vi "length_add_one.vi"(8 "error in (no error)":errorcluster, 11 "DoublyLinkedList in":refnum<class "DoublyLinkedList.lvclass">) -> (0 "error out":errorcluster, 3 "DoublyLinkedList out":refnum<class "DoublyLinkedList.lvclass">)   [LabVIEW 2021, in "DoublyLinkedList.lvclass"]
uses:
  DoublyLinkedList.lvclass
  DoublyLinkedList.lvclass/DoublyLinkedList.ctl
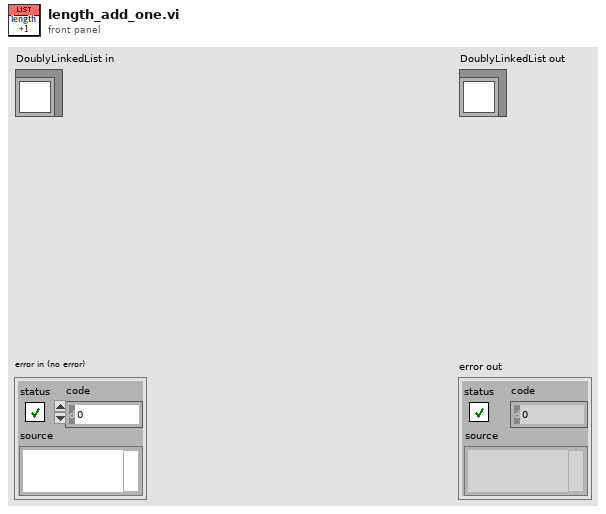
[diagram p1: front panel]
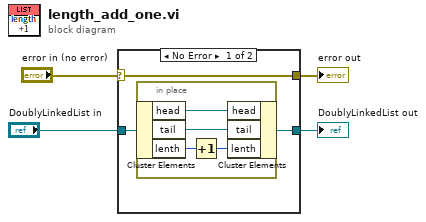
[diagram p0: block diagram]
diagram:
  n1 = case shown="No Error" "error in (no error)" {
    selector: "error in (no error)" -> [w7 w13]
    tunnel: [w7 w13] -> w3
    tunnel: [w5 w12] -> w1
    tunnel: "DoublyLinkedList in" -> [w6 w12]
    frame No Error {
      n2 = in-place {
        n3 = in-place-cluster #1(w6) -> ("head"=w8:refnum<class "DoublyNodeRef.lvclass">, "tail"=w9:refnum<class "DoublyNodeRef.lvclass">, "lenth"=w11:u32)
        n4 = Increment(x=w11) -> (x+1=w10:u32)
        n5 = in-place-cluster #1("head"=w8, "tail"=w9, "lenth"=w10) -> (w5:refnum<class "DoublyLinkedList.lvclass">)
      }
    }
    frame Error {
    }
  }
  "error out" <- w3
  "DoublyLinkedList out" <- w1
